vi "VNA - Major Cal Dual Port.vi"(0 "Cal Settings":T1={"VNA"="5632_0", "port list"="port1", "AutoCal Box Communication Port"="COM4", "Sweep Frequency Stop"=50000000.0, "Sweep Frequency Start"=50000000.0, "Output Power"=10.0, "IF Bandwidth"=100.0, "Averaging Count"=1, "Sweep Number of Points"=1, "Autocal char data file"=path "Q:/SanJose/#Karl Files/Releases/All_VNA_Calibrations/ModuleCKLab_A15080003.ACD", "Save Cal File Path"=path "C:/Calibration Files/CK Calibration - MEMS_SWITCH_50MHz.chx"} {"IF Bandwidth" format="%#_13g"; "Output Power" format="%#_13g"; "Sweep Frequency Start" format="%#_13g"; "Sweep Frequency Stop" format="%#_13g"}, 11 "error in":errorcluster {"code" format="%.0x"}) -> (4 "state":i32(ring) items=["Uncalibrated", "Calibrating", "Calibrated"], 15 "error out":errorcluster {"code" format="%.0x"})   [LabVIEW 2013]
uses:
  <instrlib>/niVNA/niVNA.llb/niVNA Perform Calibration Action (SOLT).vi
  <instrlib>/niVNA/niVNA.llb/niVNA Save Calibration And Configuration Data To File.vi
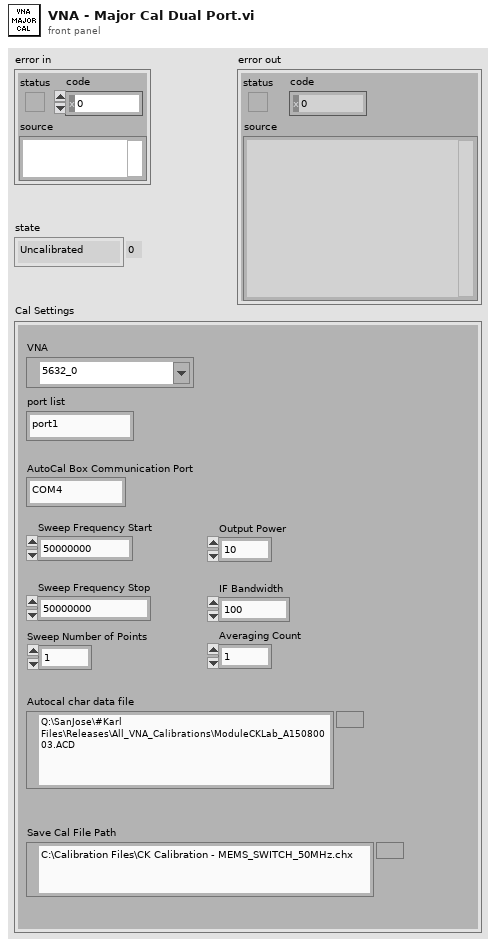
[diagram p1: front panel]
types:
  T1 = cluster{"VNA":refnum<k15>, "port list":string, "AutoCal Box Communication Port":string, "Sweep Frequency Stop":dbl, "Sweep Frequency Start":dbl, "Output Power":dbl, "IF Bandwidth":dbl, "Averaging Count":i32, "Sweep Number of Points":i32, "Autocal char data file":path, "Save Cal File Path":path}
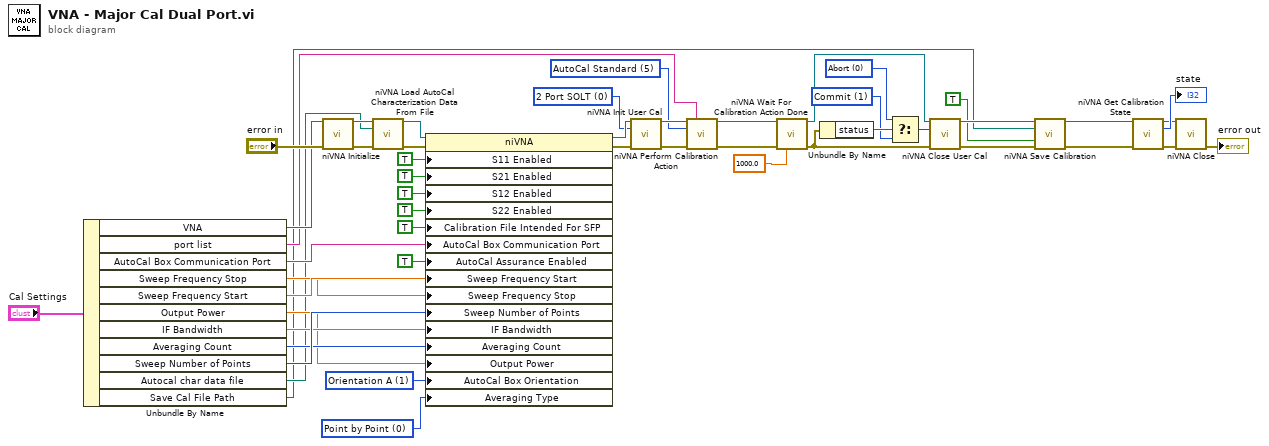
[diagram p0: block diagram]
diagram:
  w16 = 0 items=["Point by Point", "Sweep by Sweep"] ("Averaging And Smoothing:Averaging Type")
  w19 = 1 items=["Auto Sense"=2, "Orientation A"=1, "Orientation B"=0] ("Calibration Settings:AutoCal:AutoCal Box Orientation")
  w25 = 0 items=["Abort", "Commit"] ("Action")
  w23 = 1 items=["Abort", "Commit"] ("Action")
  w32 = 5 items=["Open", "Short", "Load", "Thru", "Isolation", "AutoCal Standard", "AutoCal True Thru"] ("action type")
  w33 = 0 items=["2 Port SOLT", "1 Port SOL", "Reflection Response", "Transmission Response", "TRL", "Power", "Adapter Removal"] ("calibration type")
  n1 = Unbundle By Name("Cal Settings") -> ("VNA"=w7:refnum<k15>, "port list"=w6:string, "AutoCal Box Communication Port"=w14:string, "Sweep Frequency Stop"=w12:dbl, "Sweep Frequency Start"=w13:dbl, "Output Power"=w8:dbl, "IF Bandwidth"=w10:dbl, "Averaging Count"=w9:i32, "Sweep Number of Points"=w11:i32, "Autocal char data file"=w5:path, "Save Cal File Path"=w4:path)
  n2 = call <instrlib>:"niVNA Initialize.vi"("resource name"=w7, "error in"="error in") -> ("instrument handle"=w48:refnum<k15>, "error out"=w47:errorcluster)  [unwired: 12 in]
  n3 = call <instrlib>:"niVNA Load AutoCal Characterization Data From File.vi"("instrument handle"=w48, "file path"=w5, "error in"=w47) -> ("instrument handle out"=w42:refnum<k15>, "error out"=w40:errorcluster)  [unwired: 11 in]
  n4 = property class="niVNA"(reference=w42, error in=w40, "S11 Enabled"=TRUE ("Sweep:S11 Enabled"), "S21 Enabled"=TRUE ("Sweep:S21 Enabled"), "S12 Enabled"=TRUE ("Sweep:S12 Enabled"), "S22 Enabled"=TRUE ("Sweep:S22 Enabled"), "Calibration File Intended For SFP"=TRUE ("Calibration Settings:Calibration File Intended For SFP"), "AutoCal Box Communication Port"=w14, "AutoCal Assurance Enabled"=TRUE ("Calibration Settings:AutoCal:AutoCal Assurance Enabled"), "Sweep Frequency Start"=w13, "Sweep Frequency Stop"=w12, "Sweep Number of Points"=w11, "IF Bandwidth"=w10, "Averaging Count"=w9, "Output Power"=w8, "AutoCal Box Orientation"=w19, "Averaging Type"=w16) -> (reference out=w41:refnum<k15>, error out=w39:errorcluster)
  n5 = call <instrlib>:"niVNA Init User Cal.vi"("instrument handle"=w41, "calibration type"=w33, "error in"=w39) -> ("instrument handle out"=w46:refnum<k15>, "error out"=w45:errorcluster)  [unwired: 11 in]
  n6 = call-poly <instrlib>:"niVNA Perform Calibration Action.vi"("instrument handle"=w46, "port list"=w6, "action type"=w32, "error in"=w45) -> ("instrument handle out"=w44:refnum<k15>, "error out"=w43:errorcluster)  [unwired: 10 in]
  n7 = call <instrlib>:"niVNA Wait For Calibration Action Done.vi"("instrument handle"=w44, "error in"=w43, "timeout"=1000.0) -> ("instrument handle out"=w31:refnum<k15>, "error out"=w21:errorcluster)  [unwired: 11 in]
  n8 = Unbundle By Name(w21) -> ("status"=w24:bool)
  n9 = Select(t=w25, s=w24, f=w23) -> (s? t:f=w22:i32)
  n10 = call <instrlib>:"niVNA Close User Cal.vi"("instrument handle"=w31, "action"=w22, "error in"=w21) -> ("instrument handle out"=w30:refnum<k15>, "error out"=w28:errorcluster)  [unwired: 11 in]
  n11 = call-poly <instrlib>:"niVNA Save Calibration.vi"("instrument handle"=w30, "file path"=w4, "overwrite"=TRUE, "error in"=w28) -> ("instrument handle out"=w29:refnum<k15>, "error out"=w27:errorcluster)  [unwired: 10 in]
  n12 = call <instrlib>:"niVNA Get Calibration State.vi"("instrument handle"=w29, "error in"=w27) -> ("instrument handle out"=w1:refnum<k15>, "state"=→"state":i32, "error out"=w3:errorcluster)  [unwired: 11 in]
  n13 = call <instrlib>:"niVNA Close.vi"("instrument handle"=w1, "error in"=w3) -> ("error out"=→"error out":errorcluster)  [unwired: 13 in]
